vi "Check Floors.vi"(1 "Direction":i32, 2 "Bottom":dbl, 3 "Left":dbl) -> (0 "Boolean":bool)   [LabVIEW 2014]
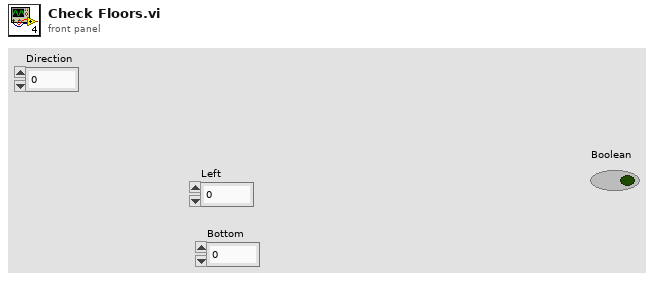
[diagram p1: front panel]
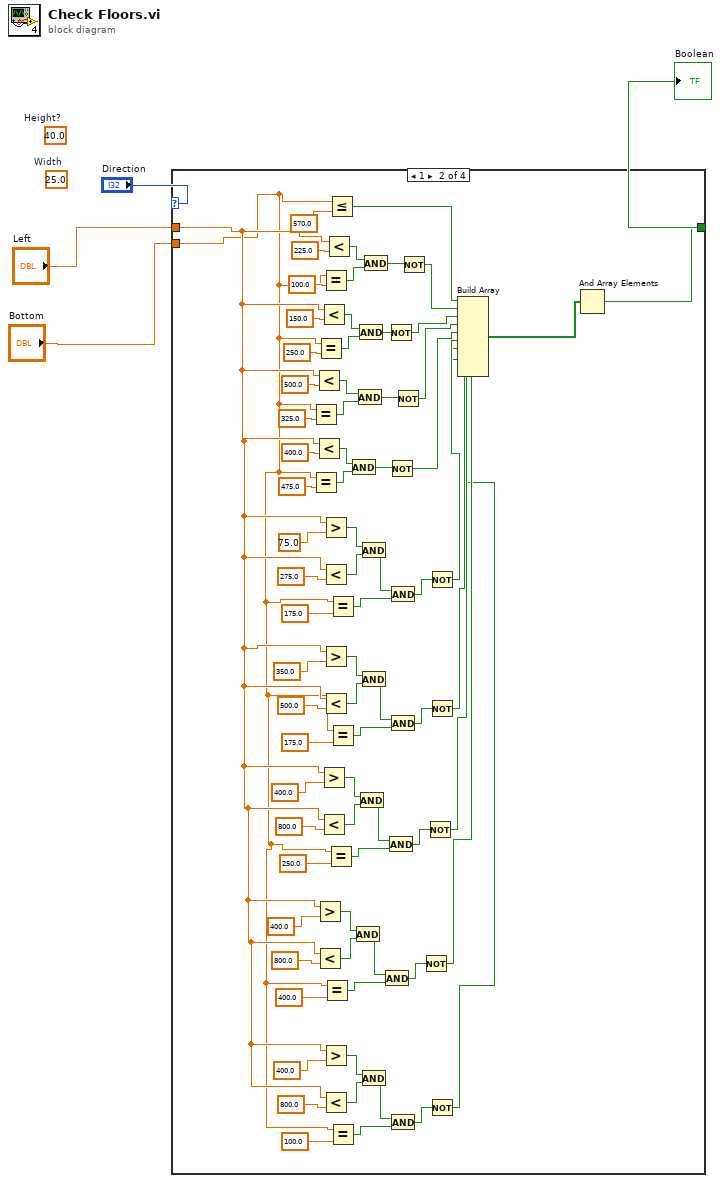
[diagram p0: block diagram]
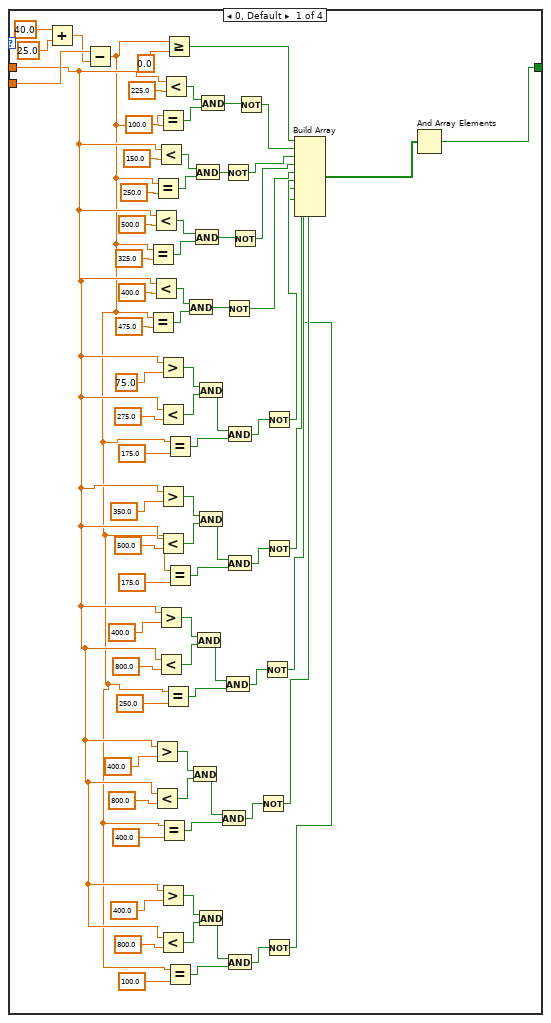
[diagram p2: hidden frame]
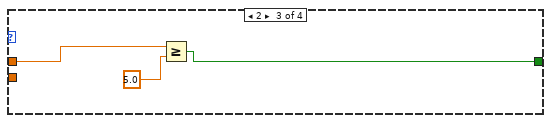
[diagram p3: hidden frame]
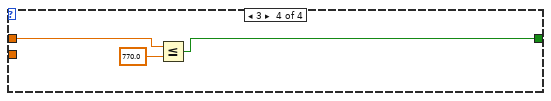
[diagram p4: hidden frame]
diagram:
  (unwired) 25.0  # Width
  (unwired) 40.0  # Height?
  n1 = case shown="1" "Direction" {
    tunnel: "Bottom" -> [w55 w84 _ _]
    tunnel: [w74 w149 w160 w163] -> w3
    tunnel: "Left" -> [w7 w86 w159 w162]
    frame 0, Default {
      n2 = Add(x=40.0 ("y"), y=25.0) -> (x+y=w53:dbl)
      n3 = Subtract(x=w55, y=w53) -> (x-y=w6:dbl)
      n4 = Equal?(x=w6, y=325.0) -> (x = y?=w62:bool)
      n5 = Equal?(x=w6, y=475.0) -> (x = y?=w59:bool)
      n6 = Less?(x=w7, y=500.0) -> (x < y?=w63:bool)
      n7 = Less?(x=w7, y=400.0) -> (x < y?=w60:bool)
      n8 = Greater?(x=w7, y=400.0) -> (0:w21:bool)
      n9 = Less?(x=w7, y=800.0) -> (x < y?=w20:bool)
      n10 = Equal?(x=w6, y=250.0) -> (x = y?=w65:bool)
      n11 = Less?(x=w7, y=150.0) -> (x < y?=w66:bool)
      n12 = Greater?(x=w7, y=400.0) -> (0:w30:bool)
      n13 = Less?(x=w7, y=800.0) -> (x < y?=w29:bool)
      n14 = Equal?(x=w6, y=100.0) -> (x = y?=w70:bool)
      n15 = Greater?(x=w7, y=75.0) -> (0:w48:bool)
      n16 = Less?(x=w7, y=275.0) -> (x < y?=w47:bool)
      n17 = Greater?(x=w7, y=350.0) -> (0:w39:bool)
      n18 = Less?(x=w7, y=500.0) -> (x < y?=w38:bool)
      n19 = Greater?(x=w7, y=400.0) -> (0:w12:bool)
      n20 = Less?(x=w7, y=800.0) -> (x < y?=w11:bool)
      n21 = Equal?(x=w6, y=400.0) -> (x = y?=w19:bool)
      n22 = Less?(x=w7, y=225.0) -> (x < y?=w71:bool)
      n23 = Equal?(x=w6, y=250.0) -> (x = y?=w28:bool)
      n24 = Greater Or Equal?(x=w6, y=0.0) -> (x >= y?=w72:bool)
      n25 = Equal?(x=w6, y=175.0) -> (x = y?=w46:bool)
      n26 = Equal?(x=w6, y=175.0) -> (x = y?=w37:bool)
      n27 = Equal?(x=w6, y=100.0) -> (x = y?=w10:bool)
      n28 = And(x=w60, y=w59) -> (x .and. y?=w61:bool)
      n29 = And(x=w21, y=w20) -> (x .and. y?=w18:bool)
      n30 = And(x=w63, y=w62) -> (x .and. y?=w64:bool)
      n31 = And(x=w66, y=w65) -> (x .and. y?=w67:bool)
      n32 = And(x=w30, y=w29) -> (x .and. y?=w27:bool)
      n33 = And(x=w48, y=w47) -> (x .and. y?=w45:bool)
      n34 = And(x=w39, y=w38) -> (x .and. y?=w36:bool)
      n35 = And(x=w12, y=w11) -> (x .and. y?=w9:bool)
      n36 = And(x=w71, y=w70) -> (x .and. y?=w69:bool)
      n37 = And(x=w18, y=w19) -> (x .and. y?=w17:bool)
      n38 = Not(x=w67) -> (.not. x?=w58:bool)
      n39 = And(x=w27, y=w28) -> (x .and. y?=w26:bool)
      n40 = Not(x=w61) -> (.not. x?=w56:bool)
      n41 = And(x=w45, y=w46) -> (x .and. y?=w44:bool)
      n42 = And(x=w36, y=w37) -> (x .and. y?=w35:bool)
      n43 = And(x=w9, y=w10) -> (x .and. y?=w8:bool)
      n44 = Not(x=w64) -> (.not. x?=w57:bool)
      n45 = Not(x=w69) -> (.not. x?=w68:bool)
      n46 = Not(x=w17) -> (.not. x?=w16:bool)
      n47 = Not(x=w26) -> (.not. x?=w25:bool)
      n48 = Not(x=w44) -> (.not. x?=w43:bool)
      n49 = Not(x=w35) -> (.not. x?=w34:bool)
      n50 = Not(x=w8) -> (.not. x?=w5:bool)
      n51 = Build Array(w72, w68, w58, w57, w56, w43, w34, w25, w16, w5) -> (w73:bool[])
      n52 = And Array Elements(Boolean array=w73) -> (logical AND=w74:bool)
    }
    frame 1 {
      n53 = Equal?(x=w84, y=325.0) -> (x = y?=w137:bool)
      n54 = Equal?(x=w84, y=475.0) -> (x = y?=w134:bool)
      n55 = Less?(x=w86, y=500.0) -> (x < y?=w138:bool)
      n56 = Less?(x=w86, y=400.0) -> (x < y?=w135:bool)
      n57 = Greater?(x=w86, y=400.0) -> (0:w100:bool)
      n58 = Less?(x=w86, y=800.0) -> (x < y?=w99:bool)
      n59 = Equal?(x=w84, y=250.0) -> (x = y?=w140:bool)
      n60 = Less?(x=w86, y=150.0) -> (x < y?=w141:bool)
      n61 = Greater?(x=w86, y=400.0) -> (0:w109:bool)
      n62 = Less?(x=w86, y=800.0) -> (x < y?=w108:bool)
      n63 = Equal?(x=w84, y=100.0) -> (x = y?=w145:bool)
      n64 = Greater?(x=w86, y=75.0) -> (0:w127:bool)
      n65 = Less?(x=w86, y=275.0) -> (x < y?=w126:bool)
      n66 = Greater?(x=w86, y=350.0) -> (0:w118:bool)
      n67 = Less?(x=w86, y=500.0) -> (x < y?=w117:bool)
      n68 = Greater?(x=w86, y=400.0) -> (0:w91:bool)
      n69 = Less?(x=w86, y=800.0) -> (x < y?=w90:bool)
      n70 = Equal?(x=w84, y=400.0) -> (x = y?=w98:bool)
      n71 = Less?(x=w86, y=225.0) -> (x < y?=w146:bool)
      n72 = Equal?(x=w84, y=250.0) -> (x = y?=w107:bool)
      n73 = Less Or Equal?(x=w84, y=570.0) -> (x <= y?=w147:bool)
      n74 = Equal?(x=w84, y=175.0) -> (x = y?=w125:bool)
      n75 = Equal?(x=w84, y=175.0) -> (x = y?=w116:bool)
      n76 = Equal?(x=w84, y=100.0) -> (x = y?=w89:bool)
      n77 = And(x=w135, y=w134) -> (x .and. y?=w136:bool)
      n78 = And(x=w100, y=w99) -> (x .and. y?=w97:bool)
      n79 = And(x=w138, y=w137) -> (x .and. y?=w139:bool)
      n80 = And(x=w141, y=w140) -> (x .and. y?=w142:bool)
      n81 = And(x=w109, y=w108) -> (x .and. y?=w106:bool)
      n82 = And(x=w127, y=w126) -> (x .and. y?=w124:bool)
      n83 = And(x=w118, y=w117) -> (x .and. y?=w115:bool)
      n84 = And(x=w91, y=w90) -> (x .and. y?=w88:bool)
      n85 = And(x=w146, y=w145) -> (x .and. y?=w144:bool)
      n86 = And(x=w97, y=w98) -> (x .and. y?=w96:bool)
      n87 = Not(x=w142) -> (.not. x?=w133:bool)
      n88 = And(x=w106, y=w107) -> (x .and. y?=w105:bool)
      n89 = Not(x=w136) -> (.not. x?=w131:bool)
      n90 = And(x=w124, y=w125) -> (x .and. y?=w123:bool)
      n91 = And(x=w115, y=w116) -> (x .and. y?=w114:bool)
      n92 = And(x=w88, y=w89) -> (x .and. y?=w87:bool)
      n93 = Not(x=w139) -> (.not. x?=w132:bool)
      n94 = Not(x=w144) -> (.not. x?=w143:bool)
      n95 = Not(x=w96) -> (.not. x?=w95:bool)
      n96 = Not(x=w105) -> (.not. x?=w104:bool)
      n97 = Not(x=w123) -> (.not. x?=w122:bool)
      n98 = Not(x=w114) -> (.not. x?=w113:bool)
      n99 = Not(x=w87) -> (.not. x?=w85:bool)
      n100 = Build Array(w147, w143, w133, w132, w131, w122, w113, w104, w95, w85) -> (w148:bool[])
      n101 = And Array Elements(Boolean array=w148) -> (logical AND=w149:bool)
    }
    frame 2 {
      n102 = Greater Or Equal?(x=w159, y=5.0) -> (x >= y?=w160:bool)
    }
    frame 3 {
      n103 = Less Or Equal?(x=w162, y=770.0) -> (x <= y?=w163:bool)
    }
  }
  "Boolean" <- w3
